vi "PhysMon-Select Output Filename.vi"(0 "File":path, 11 "error in (no error)":errorcluster) -> (4 "File Out":path, 8 "Continue?":bool, 15 "error out":errorcluster)   [LabVIEW 2020]
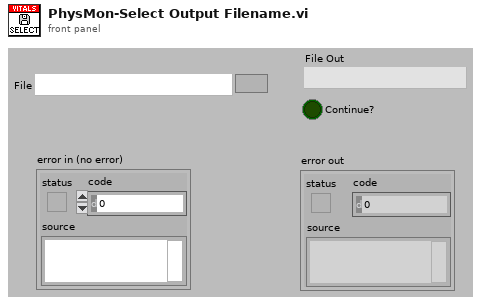
[diagram p1: front panel]
types:
  T1 = enum16{"Left Button", "Center Button", "Right Button", "Window Close"}
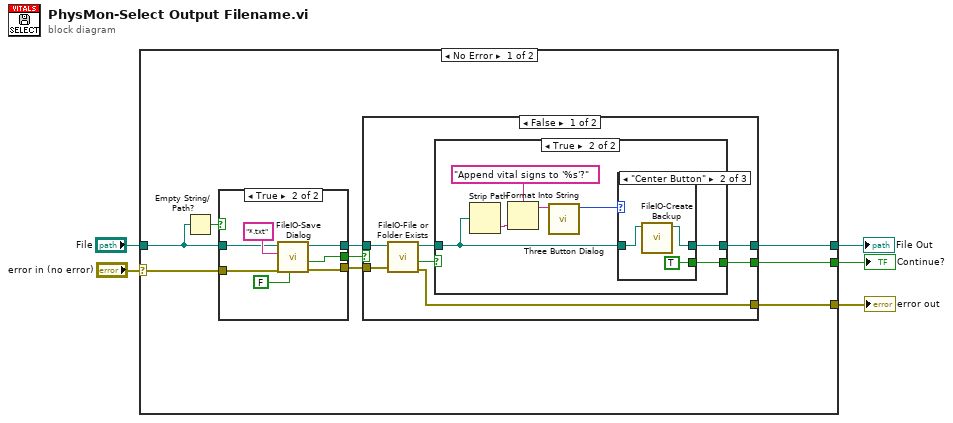
[diagram p0: block diagram]
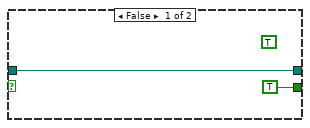
[diagram p2: hidden frame]
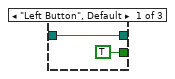
[diagram p3: hidden frame]
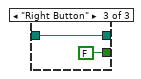
[diagram p4: hidden frame]
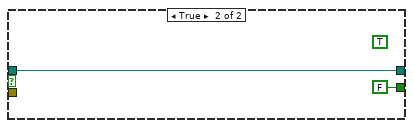
[diagram p5: hidden frame]
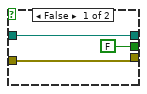
[diagram p6: hidden frame]
diagram:
  n1 = case shown="No Error" "error in (no error)" {
    selector: "error in (no error)" -> [w13 w50]
    tunnel: [w10 w50] -> w4
    tunnel: "File" -> [w14 _]
    tunnel: [w12 _] -> w2
    tunnel: [w11 _] -> w1
    frame No Error {
      n2 = Empty String/Path?(string/path=w14) -> (empty?=w9:bool)
      n3 = case shown="True" w9 {
        tunnel: w14 -> [w42 w48]
        tunnel: [w42 w47] -> w8
        tunnel: [FALSE w43] -> w6
        tunnel: w13 -> [w40 w46]
        tunnel: [w40 w45] -> w7
        frame False {
        }
        frame True {
          n4 = call "FileIO-Save Dialog.vi"("Overwrite prompt?"=FALSE, "error in"=w46, "pattern (all files)"="*.txt", "Start path"=w48) -> ("error out"=w45:errorcluster, "cancelled"=w43:bool, "selected path"=w47:path)  [unwired: 5 in]
        }
      }
      n5 = case shown="False" w6 {
        tunnel: w8 -> [w19 w39]
        tunnel: w7 -> [w18 _]
        tunnel: [w16 FALSE] -> w11
        tunnel: [w17 w39] -> w12
        tunnel: [w15 _] -> w10
        frame False {
          n6 = call "FileIO-File or Folder Exists.vi"("error in (no error)"=w18, "path"=w19) -> ("error out"=w15:errorcluster, "Exists?"=w21:bool, "dup path"=w20:path)  [unwired: 6 in, 1 out]
          n7 = case shown="True" w21 {
            tunnel: w20 -> [w23 w25]
            tunnel: [w23 w24] -> w17
            tunnel: [TRUE w26] -> w16
            frame False {
              (unwired) TRUE
            }
            frame True {
              n8 = Strip Path(path=w25) -> (name=w29:string)  [unwired: 1 out]
              n9 = Format Into String(format string="Append vital signs to '%s'?" ("message"), w29) -> (resulting string=w28:string)  [unwired: 2 in, 1 out]
              n10 = call <vilib>:"Three Button Dialog.vi"("message"=w28) -> ("Which Button?"=w27:T1)  [unwired: 10 in]
              n11 = case shown="\"Center Button\"" w27 {
                tunnel: [TRUE TRUE FALSE] -> w26
                tunnel: w25 -> [w31 w34 w36]
                tunnel: [w31 w33 w36] -> w24
                frame "Left Button", Default {
                }
                frame "Center Button" {
                  n12 = call "FileIO-Create Backup.vi"("Path"=w34) -> ("Path (thru)"=w33:path)  [unwired: 7 in, 3 out]
                }
                frame "Right Button" {
                }
              }
            }
          }
        }
        frame True {
          (unwired) TRUE
        }
      }
    }
    frame Error {
    }
  }
  "error out" <- w4
  "File Out" <- w2
  "Continue?" <- w1
